vi "SVFA Convert Spectrum X Units.vi"   [LabVIEW 2017]
doc: "Converts a frequency power spectrum to an order power spectrum. Use this VI to convert power spectrum results from constant-speed applications."
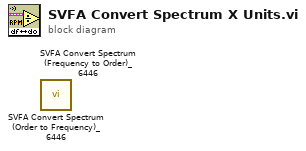
[diagram p0: block diagram]
diagram:
  n1 = call <vilib>:"SVFA Convert Spectrum (Order to Frequency)_6446.vi"() -> ()  [unwired: 18 in, 2 out]
  n2 = call <vilib>:"SVFA Convert Spectrum (Frequency to Order)_6446.vi"() -> ()  [unwired: 18 in, 2 out]
